vi "S2DS_Edit external instrument.vi"(8 "error in (no error)":errorcluster, 11 "Instrument parameters in":T1) -> (0 "error out":errorcluster, 3 "Instrument parameters out":T1)   [LabVIEW 2025]
panel:
  in  "Max Wait Time (ms)":i32
  in  "Precison":dbl
  in  "Wait?":bool caption="Wait and check for \ntarget to be set?"
  in  "Update?":bool
  # "External instrument settings"
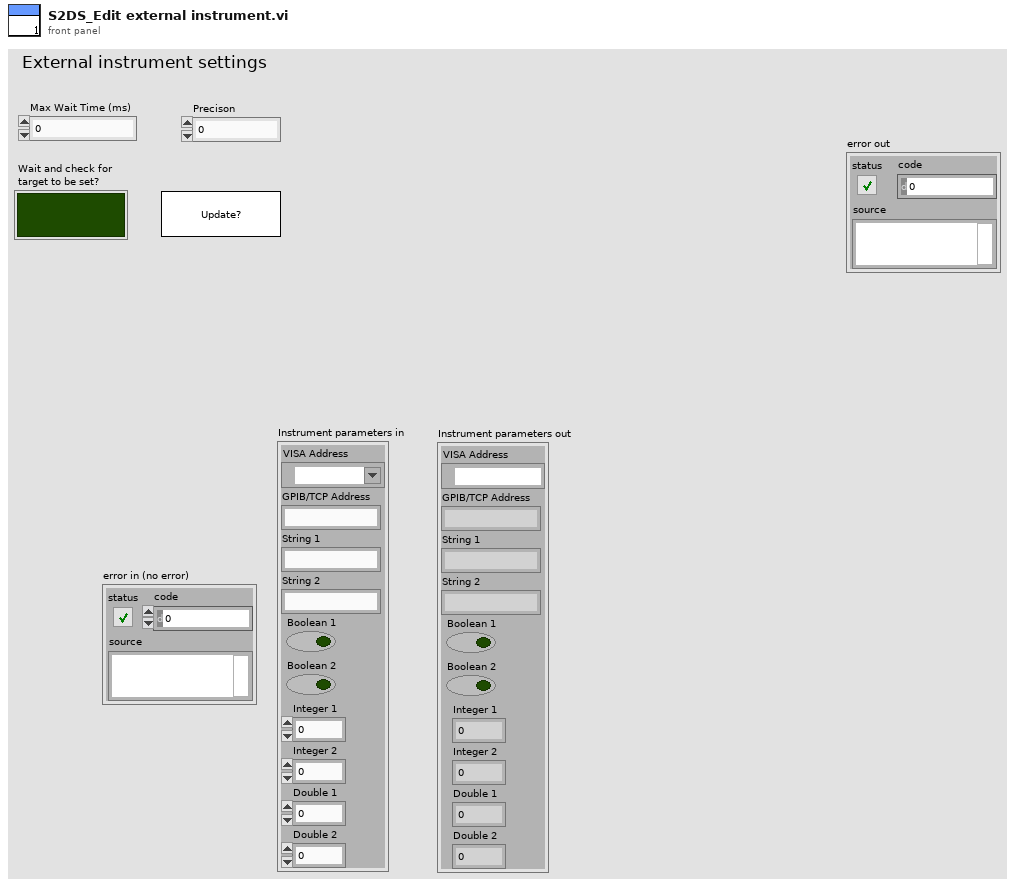
[diagram p1: front panel]
types:
  T1 = cluster{"VISA Address":refnum<visa-resource-name>, "GPIB/TCP Address":string, "String 1":string, "String 2":string, "Boolean 1":bool, "Boolean 2":bool, "Integer 1":i32, "Integer 2":i32, "Double 1":dbl, "Double 2":dbl}
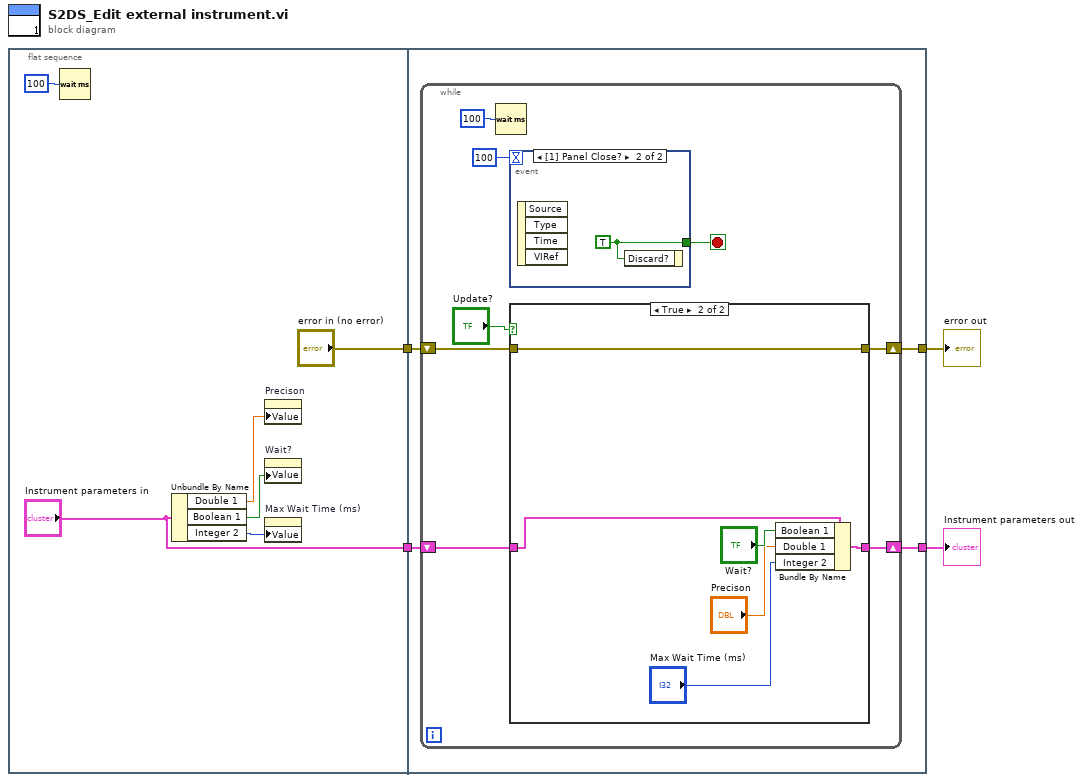
[diagram p0: block diagram]
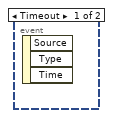
[diagram p3: hidden frame]
diagram:
  n1 = flat-sequence {
    tunnel: ["Instrument parameters in"] -> w4
    tunnel: ["error in (no error)"] -> w2
    tunnel: w4 -> [w14]
    tunnel: [w13] -> w3
    tunnel: w2 -> [w12]
    tunnel: [w11] -> w1
    frame #0 {
      n2 = Wait (ms)(milliseconds to wait=u32 100) -> ()  [unwired: 1 out]
      n3 = Unbundle By Name("Instrument parameters in") -> ("Double 1"=w7:dbl, "Boolean 1"=w6:bool, "Integer 2"=w5:i32)
      n4 = property on="Precison" class="DigNum (strict)"("Value"=w7) -> ()  [unwired: 2 in, 2 out]
      n5 = property on="Wait?" class="Bool (strict)"("Value"=w6) -> ()  [unwired: 2 in, 2 out]
      n6 = property on="Max Wait Time (ms)" class="DigNum (strict)"("Value"=w5) -> ()  [unwired: 2 in, 2 out]
    }
    frame #1 {
      n7 = while {
        shift-right: [w21] -> w13
        shift-left: w14 -> [w16]
        shift-right: [w18] -> w11
        shift-left: w12 -> [w15]
        stop <- w20 stop-if-true
        n8 = Wait (ms)(milliseconds to wait=u32 100) -> ()  [unwired: 1 out]
        n9 = event shown="[1] Panel Close?" {
          selector: _ -> [_ _]
          dyn-events: _ -> [_ _]
          timeout: 100 -> [_ _]
          tunnel: [_ w31] -> w20
          event Timeout {
            n10 = event-data() -> ()  [unwired: 1 in, 3 out]
          }
          event Panel Close? {
            w31 = TRUE ("Discard?")
            n11 = event-data() -> ()  [unwired: 1 in, 4 out]
            n12 = event-data("Discard?"=w31) -> ()  [unwired: 1 in, 1 out]
          }
        }
        n13 = case shown="True" "Update?" {
          tunnel: [w24 w29] -> w21
          tunnel: [w23 w28] -> w18
          tunnel: w16 -> [w24 w30]
          tunnel: w15 -> [w23 w28]
          frame False {
          }
          frame True {
            n14 = Bundle By Name(cluster=w30, "Boolean 1"="Wait?", "Double 1"="Precison", "Integer 2"="Max Wait Time (ms)") -> (w29:T1)
          }
        }
      }
    }
  }
  "Instrument parameters out" <- w3
  "error out" <- w1
